vi "FTW-JSON-Object-SetElement-String.vi"(0 "JSON Object":refnum<data-value>, 5 "Key":string, 7 "Value":string, 11 "error in":errorcluster) -> (4 "JSON Object out":refnum<data-value>, 15 "error out":errorcluster)   [LabVIEW 2014]
uses:
  core/FTW-JSON-Core-Structure.ctl
  error/FTW-ERR-ThrowGenericError.vi
  error/FTW-ERR-ThrowError.vi
  error/FTW-ERR-NoErrorConstant.vi
  error/FTW-ERR-CallChain.vi
  string/FTW-STR-ReplaceWhitespace.vi
panel:
  # "Inputs"
  # "Outputs"
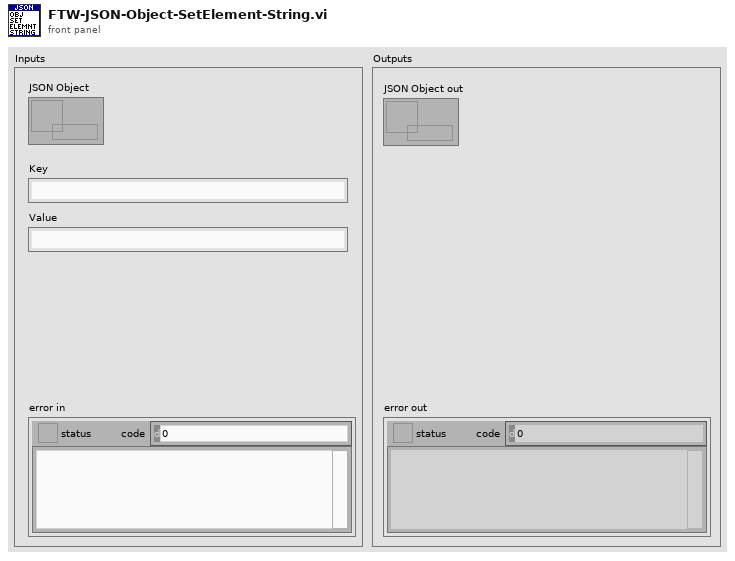
[diagram p1: front panel]
types:
  T1 = typedef "FTW-JSON-Core-Structure.ctl" = cluster{"JSON Object":i64, "Encoding Flags":i64, "Decoding Flags":i64}
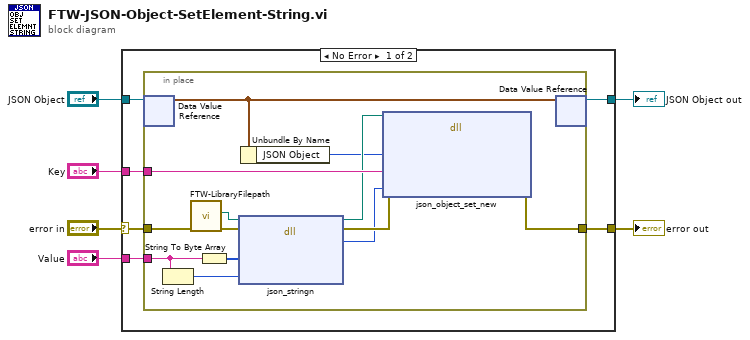
[diagram p0: block diagram]
diagram:
  n1 = case shown="No Error" "error in" {
    selector: "error in" -> [w12 w27]
    tunnel: [w11 w27] -> w6
    tunnel: [w7 w26] -> w4
    tunnel: "JSON Object" -> [w8 w26]
    tunnel: "Key" -> [w10 _]
    tunnel: "Value" -> [w9 _]
    frame No Error {
      n2 = in-place {
        in-place-border: w12 -> [w25]
        in-place-border: [w24] -> w11
        in-place-border: w10 -> [w23]
        in-place-border: w9 -> [w18]
        n3 = in-place-dvr #1(w8) -> (w15:T1)  [unwired: 1 out]
        n4 = String Length(string=w18) -> (length=w17:i32)
        n5 = call "FTW-LibraryFilepath.vi"("error in"=w25) -> ("error out"=w20:errorcluster, "Library Filepath"=w22:path)  [unwired: 8 in, 1 out]
        n6 = String To Byte Array(string=w18) -> (unsigned byte array=w13:u8[])
        n7 = dll-call lib="?" fn="json_stringn"(path in=w22, error in=w20, "String Value"=w13, "String Length"=w17) -> (path out=w21:path, error out=w19:errorcluster, "New String Value"=w16:i64)  [unwired: 3 in]
        n8 = Unbundle By Name(w15) -> ("JSON Object"=w14:i64)
        n9 = dll-call lib="?" fn="json_object_set_new"(path in=w21, error in=w19, "JSON Object Pointer"=w14, "Key"=w23, "New JSON Object"=w16) -> (error out=w24:errorcluster)  [unwired: 5 in, 1 out]
        n10 = in-place-dvr #1(w15) -> (w7:refnum<data-value>)  [unwired: 1 out]
      }
    }
    frame Error {
    }
  }
  "error out" <- w6
  "JSON Object out" <- w4
